vi "转换为ASCII.vi"(11 "字符串":string) -> (3 "字符串 2":string)   [LabVIEW 2012]
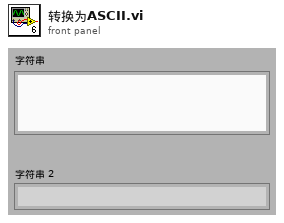
[diagram p1: front panel]
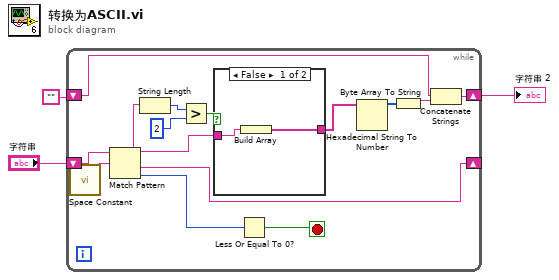
[diagram p0: block diagram]
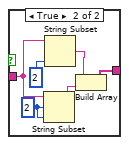
[diagram p2: hidden frame]
diagram:
  n1 = while {
    shift-right: [w16] -> _
    shift-left: "字符串" -> [w17]
    shift-right: [w11] -> w1
    shift-left: "" -> [w13]
    stop <- w9 stop-if-true
    n2 = call <vilib>:"Space Constant.vi"() -> ("String"=w15:string)
    n3 = Match Pattern(string=w17, regular expression=w15) -> (before substring=w5:string, after substring=w16:string, offset past match=w10:i32)  [unwired: 2 out]
    n4 = String Length(string=w5) -> (length=w8:i32)
    n5 = Greater?(x=w8, y=2) -> (0:w6:bool)
    n6 = case shown="False" w6 {
      tunnel: w5 -> [w19 w24]
      tunnel: [w18 w20] -> w4
      frame False {
        n7 = Build Array(w19) -> (w18:string[])
      }
      frame True {
        w23 = 2 ("偏移量(0)")
        n8 = String Subset(string=w24, offset (0)=w23, length (rest)=w23) -> (substring=w21:string)
        n9 = String Subset(string=w24, length (rest)=2 ("长度（剩余）")) -> (substring=w22:string)  [unwired: 1 out]
        n10 = Build Array(w22, w21) -> (w20:string[])
      }
    }
    n11 = Less Or Equal To 0?(x=w10) -> (x <= 0?=w9:bool)
    n12 = Hexadecimal String To Number(string=w4) -> (number=w14:u32[])  [unwired: 3 out]
    n13 = Byte Array To String(unsigned byte array=w14) -> (string=w12:string)
    n14 = Concatenate Strings(w13, w12) -> (w11:string)
  }
  "字符串 2" <- w1
